vi "exit.vi"(8 "error in (no error)":errorcluster, 11 "Model in":refnum<class "Model.lvclass">) -> (0 "error out":errorcluster, 3 "Model out":refnum<class "Model.lvclass">)   [LabVIEW 2016, in "Model.lvclass"]
uses:
  Model.lvclass
  Types/ShutdownEvent.ctl
  Model.lvclass/Model.ctl
  UserEvents/UserEvents.lvclass/UserEvents.ctl
  UserEvents/UserEvents.lvclass
  Types/M1M3SupportTypes.lvlib
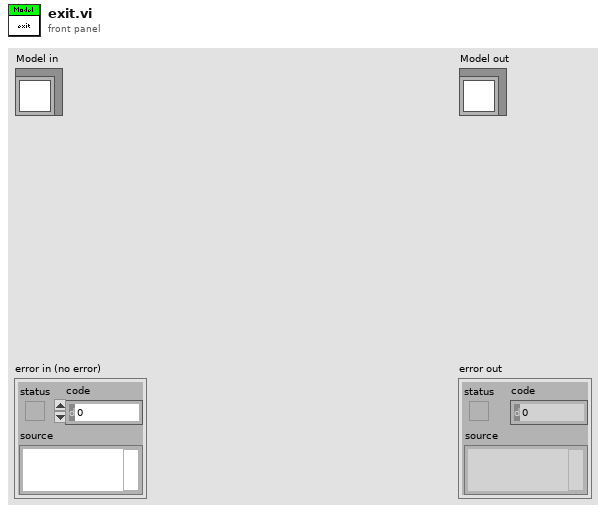
[diagram p1: front panel]
types:
  T1 = typedef "M1M3SupportTypes.lvlib/ShutdownEvent.ctl" = cluster{"Shutdown":bool}
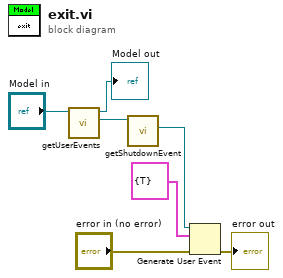
[diagram p0: block diagram]
diagram:
  n1 = call "getUserEvents.vi"("Model in"="Model in") -> ("UserEvents"=w6:refnum<class "UserEvents.lvclass">, "Model out"=→"Model out":refnum<class "Model.lvclass">)  [unwired: 9 in]
  n2 = call "getShutdownEvent.vi"("UserEvents in"=w6) -> ("ShutdownEvent"=w5:refnum<user-event>)  [unwired: 9 in, 1 out]
  n3 = Generate User Event(user event=w5, event data cluster=T1 {"Shutdown"=TRUE} ("event data"), error in="error in (no error)") -> (error out=→"error out":errorcluster)  [unwired: 1 in, 1 out]
